vi "getRoutings.vi"(8 "error in (no error)":errorcluster, 11 "DigitalDevice.lvclass in":refnum<class "DigitalDevice.lvclass">) -> (0 "error out":errorcluster, 2 "Routings":cluster{"Master Clock Route":string[]}, 3 "DigitalDevice.lvclass out":refnum<class "DigitalDevice.lvclass">)   [LabVIEW 2009, in "Tools.lvlib" / "DatabaseHelpers.lvlib" / "DigitalDevice.lvclass"]
uses:
  DigitalDevice.lvclass
  DigitalDevice.lvclass/DigitalDevice.ctl
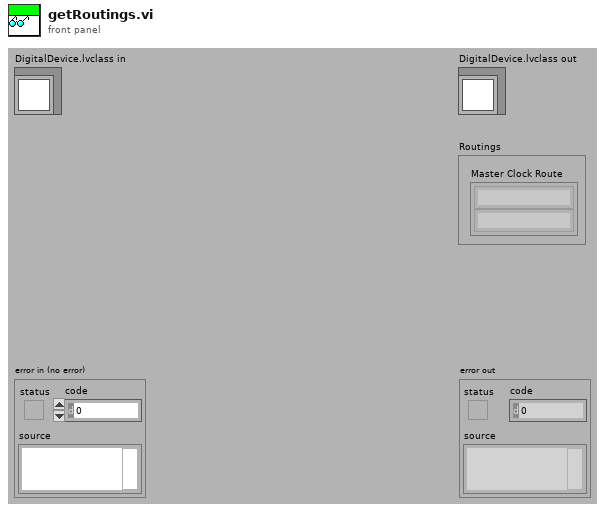
[diagram p1: front panel]
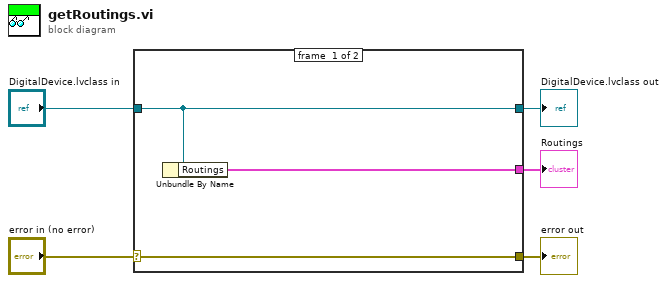
[diagram p0: block diagram]
diagram:
  n1 = case shown="No Error" "error in (no error)" {
    selector: "error in (no error)" -> [w8 w9]
    tunnel: [w8 w9] -> w4
    tunnel: [w7 w10] -> w2
    tunnel: "DigitalDevice.lvclass in" -> [w7 w10]
    tunnel: [w6 _] -> w1
    frame #0 {
      n2 = Unbundle By Name(w7) -> ("Routings"=w6:cluster{"Master Clock Route":string[]})
    }
    frame #1 {
    }
  }
  "error out" <- w4
  "DigitalDevice.lvclass out" <- w2
  "Routings" <- w1
